vi "camera acquire test.vi"() -> ()   [LabVIEW 2014]
uses:
  SubVIs/ctt's/image acquisiton 4.ctl
  SubVIs/ctt's/image acquisition 3.ctl
  <vilib>/vision/Image Controls.llb/IMAQ Image.ctl
  SubVIs/Initilize Globals.vi
  lib/Andorlib/atmcd32d.lvlib
panel:
  out "New Image":T1
  out "Actual Exposure Time (s)":dbl format="%#_13g"
  in  "High Capacity?":bool
  in  "Acquisition Parameters":T2={"Readout Mode"=enum."Image", "Set Acquisition Mode"=enum."Single Scan", "Trigger Mode"=enum."Internal", "Exposure Time (s)"=1.0, "Accumulation Cycle (s)"=1.0, "Kinetic Cycle Time (s)"=1.0, "Number of Kinetics"=1, "Number of Accumulations"=1, "Set VS Speed"=1, "Pixel Rate"=enum."Standard CCD 3 Mhz 14 bits", "V Shift Amplitude"=enum."+1", "Preamp Gain"=enum."1.0"}
  in  "Image Size":T3={"H Bin"=1024.0, "V Bin"=1024.0, "Left"=1.0, "Right"=1024.0, "Top"=1.0, "Bottom"=1024.0} {"V Bin" min=0.0; "H Bin" min=0.0 step=1.0}
  out "Error Out":errorcluster
  out "Error Return":i32
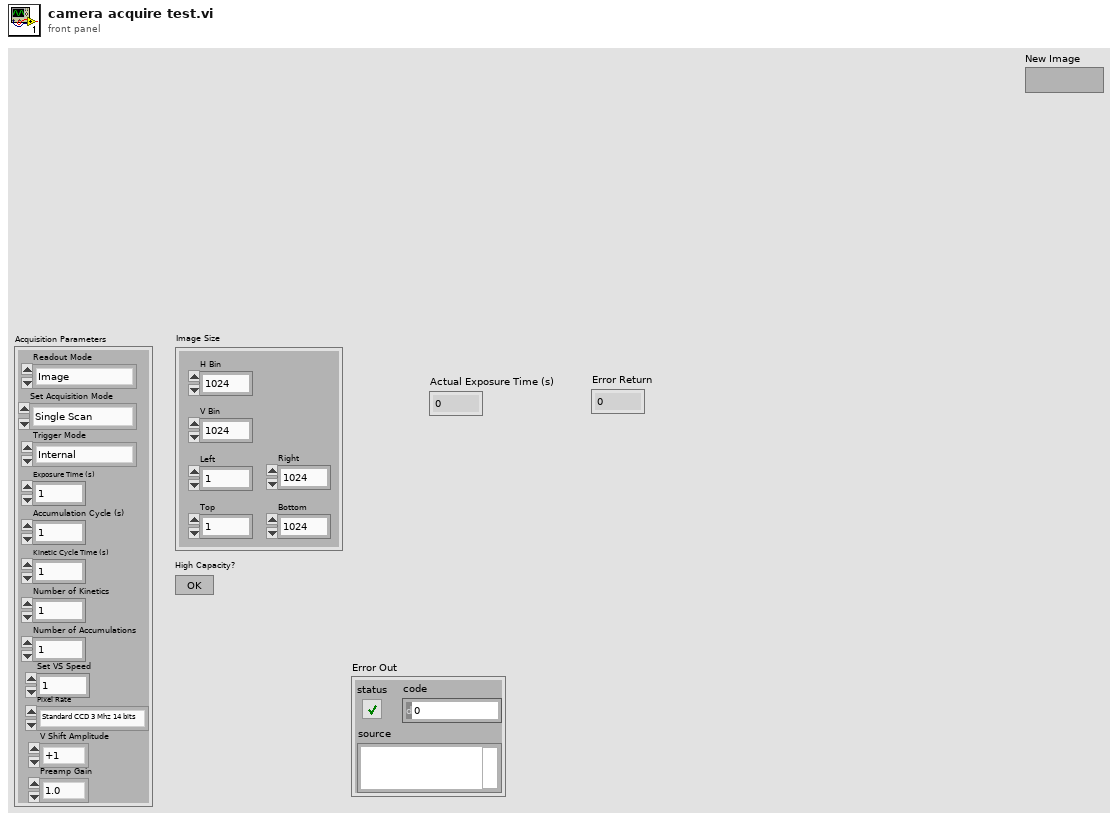
[diagram p1: front panel]
types:
  T1 = typedef "IMAQ Image.ctl" = refnum<image>
  T2 = typedef "image acquisition 3.ctl" = cluster{"Readout Mode":enum16{"Full Vertical Binning", "Multi-Track", "Random-Track", "Single-Track", "Image"}, "Set Acquisition Mode":enum16{"(do nothing)", "Single Scan", "Accumulate", "Kinetics", "Fast Kinetics", "Run till abort"}, "Trigger Mode":enum16{"Internal", "External"}, "Exposure Time (s)":dbl, "Accumulation Cycle (s)":dbl, "Kinetic Cycle Time (s)":dbl, "Number of Kinetics":i32, "Number of Accumulations":i32, "Set VS Speed":i32, "Pixel Rate":enum16{"EM CCD 10 Mhz 14 bits", "EM CCD 5 Mhz 14 bits", "EM CCD 3 Mhz 14 bits", "EM CCD 1 Mhz 16 bits", "Standard CCD 3 Mhz 14 bits", "Standard CCD 1 Mhz 16 bits"}, "V Shift Amplitude":enum16{"normal", "+1", "+2", "+3", "+4"}, "Preamp Gain":enum16{"1.0", "2.4", "5.0"}}
  T3 = typedef "image acquisiton 4.ctl" = cluster{"H Bin":dbl, "V Bin":dbl, "Left":dbl, "Right":dbl, "Top":dbl, "Bottom":dbl}
  T4 = typedef "Image Type" = u32
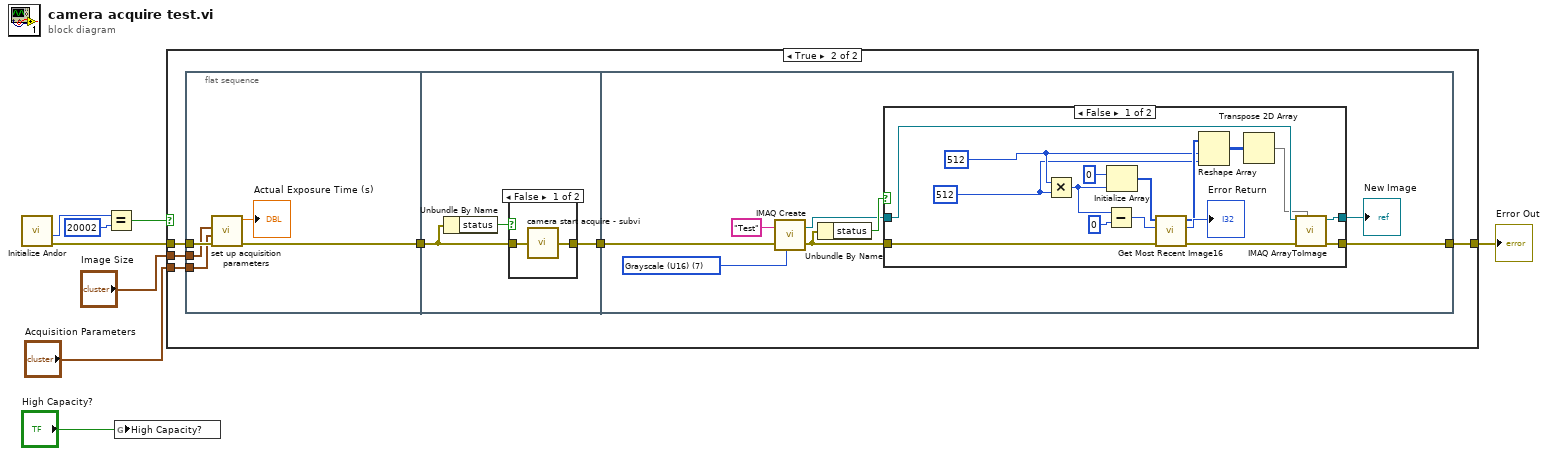
[diagram p0: block diagram]
diagram:
  n1 = call "Initialize Andor.vi"() -> ("Error Out 2"=w4:errorcluster, "Drv Success?"=w1:i32)  [unwired: 10 in]
  n2 = Equal?(x=w1, y=20002) -> (x = y?=w3:bool)
  n3 = global write "Initilize Globals.vi" "High Capacity?"("High Capacity?") -> ()
  n4 = case shown="True" w3 {
    tunnel: [w9 w13] -> w8
    tunnel: "Acquisition Parameters" -> [_ w12]
    tunnel: w4 -> [w9 w11]
    tunnel: "Image Size" -> [_ w10]
    frame False {
    }
    frame True {
      n5 = flat-sequence {
        tunnel: [w17] -> w15
        tunnel: w12 -> [w18]
        tunnel: w11 -> [w20]
        tunnel: w10 -> [w19]
        tunnel: w15 -> [w22]
        tunnel: [w21] -> w14
        tunnel: w14 -> [w31]
        tunnel: [w27] -> w13
        frame #0 {
          n6 = call "set up acquisition parameters.vi"("error in (no error)"=w20, "Acquisition Parameters"=w18, "Image Size"=w19) -> ("error out"=w17:errorcluster, "Exposure"=→"Actual Exposure Time (s)":dbl)  [unwired: 2 in, 3 out]
        }
        frame #1 {
          n7 = Unbundle By Name(w22) -> ("status"=w23:bool)
          n8 = case shown="False" w23 {
            tunnel: w22 -> [w25 w26]
            tunnel: [w24 w26] -> w21
            frame False {
              n9 = call "camera start acquire - subvi.vi"("error in"=w25) -> ("error out"=w24:errorcluster)
            }
            frame True {
            }
          }
        }
        frame #2 {
          w33 = T4 7 items=["Grayscale (U8)", "Grayscale (I16)", "Grayscale (SGL)", "Complex (CSG)", "RGB (U32)", "HSL (U32)", "RGB (U64)", "Grayscale (U16)"] ("Image Type")
          n10 = call "IMAQ Create"("Image Name"="Test", "Image Type"=w33, "error in (no error)"=w31) -> ("New Image"=w29:T1, "error out"=w28:errorcluster)  [unwired: 2 in]
          n11 = Unbundle By Name(w28) -> ("status"=w34:bool)
          n12 = case shown="False" w34 {
            tunnel: w28 -> [w50 w51]
            tunnel: w29 -> [w43 w52]
            tunnel: [w42 w52] -> w30
            tunnel: [w41 w51] -> w27
            frame False {
              w35 = 512
              w36 = 512
              n13 = Multiply(x=w36, y=w35) -> (x*y=w40:i32)
              n14 = Subtract(x=w40, y=0) -> (x-y=w38:i32)
              n15 = Initialize Array(u16 0, w40) -> (w48:u16[])
              n16 = call "Get Most Recent Image16.vi"("error in (no error)"=w50, "size"=w38, "Array 2"=w48) -> ("error out"=w44:errorcluster, "function return"=→"Error Return":u32, "Array"=w46:u16[])  [unwired: 6 in]
              n17 = Reshape Array(w46, w36, w35) -> (w45:u16[][])
              n18 = Transpose 2D Array(2D array=w45) -> (transposed array=w37:u16[][])
              n19 = call "IMAQ ArrayToImage"("Image Pixels (U16)"=w37, "error in (no error)"=w44, "Image"=w43) -> ("error out"=w41:errorcluster, "Image Out"=w42:T1)  [unwired: 3 in, 4 out]
            }
            frame True {
            }
          }
          "New Image" <- w30
        }
      }
    }
  }
  "Error Out" <- w8
